vi "Get Data Queue Values.vi"(8 "error in (no error)":errorcluster, 11 "Sift Client in":refnum<class "Sift Client.lvclass">) -> (0 "error out":errorcluster, 2 "map":map{string, variant}(c390), 3 "Sift Client out":refnum<class "Sift Client.lvclass">)   [LabVIEW 2024, in "Sift Client.lvlib" / "Sift Client.lvclass"]
uses:
  Sift Client.lvclass
  Sift Client.lvclass/Sift Client.ctl
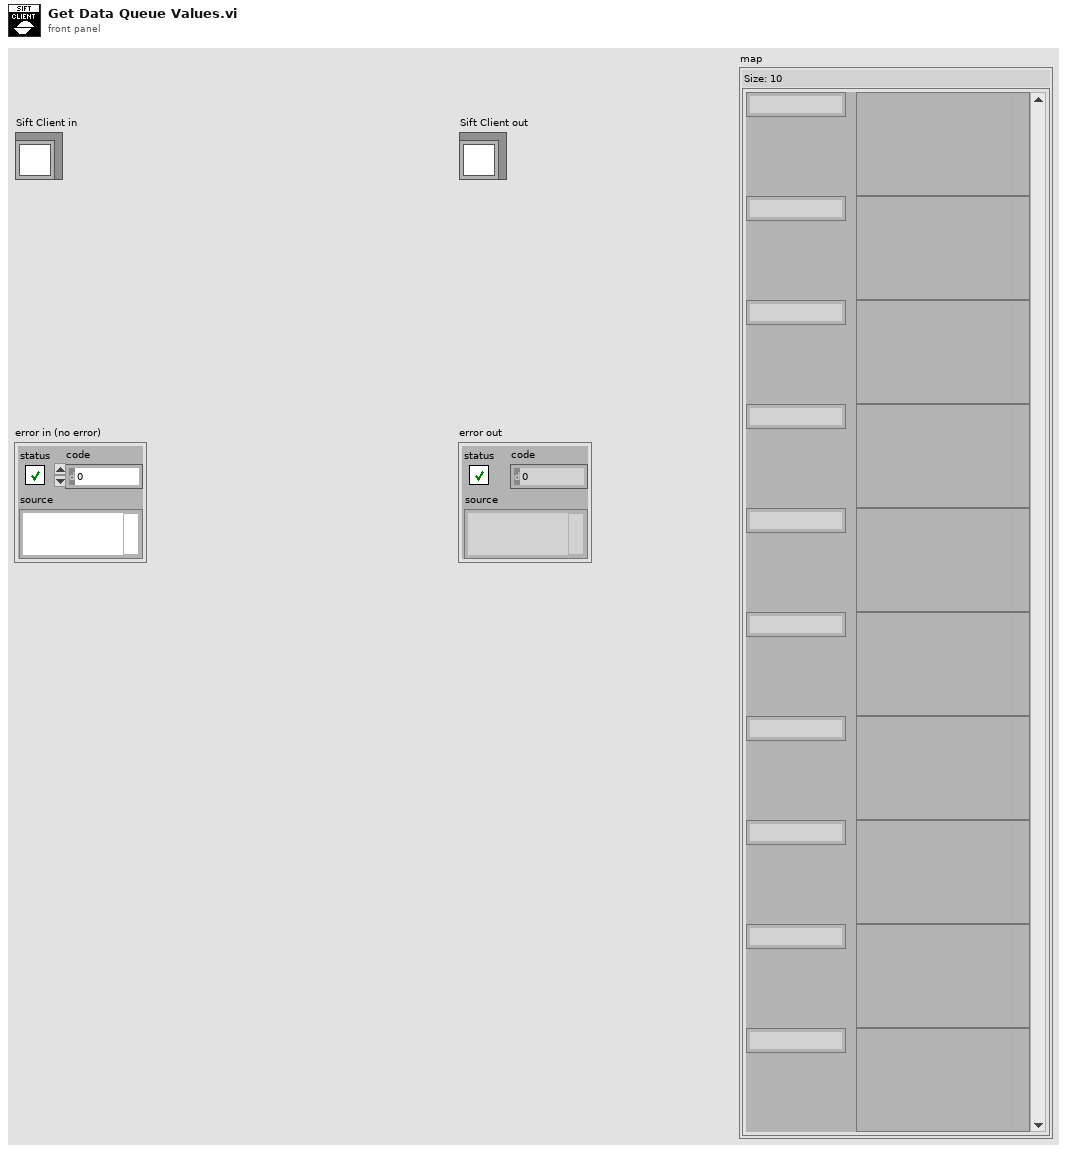
[diagram p1: front panel]
types:
  T1 = typedef "Sift Client.lvlib/String Sample.ctl" = cluster{"Values":string[], "Timestamp":T2, "Flow Name":string}
  T2 = typedef "SiftProxy_client.lvlib/google_protobuf_Timestamp.ctl" = cluster{"seconds":i64, "nanos":i32}
  T3 = typedef "Sift Client.lvlib/Double Sample.ctl" = cluster{"Values":dbl[], "Timestamp":T2, "Flow Name":string}
  T4 = typedef "Sift Client.lvlib/Float Sample.ctl" = cluster{"Values":sgl[], "Timestamp":T2, "Flow Name":string}
  T5 = typedef "Sift Client.lvlib/Int64 Sample.ctl" = cluster{"Values":i64[], "Timestamp":T2, "Flow Name":string}
  T6 = typedef "Sift Client.lvlib/Bool Sample.ctl" = cluster{"Values":bool[], "Timestamp":T2, "Flow Name":string}
  T7 = typedef "Sift Client.lvlib/Int32 Sample.ctl" = cluster{"Values":i32[], "Timestamp":T2, "Flow Name":string}
  T8 = typedef "Sift Client.lvlib/Uint64 Sample.ctl" = cluster{"Values":u64[], "Timestamp":T2, "Flow Name":string}
  T9 = typedef "Sift Client.lvlib/Uint32 Sample.ctl" = cluster{"Values":u32[], "Timestamp":T2, "Flow Name":string}
  T10 = typedef "Sift Client.lvlib/Enum Sample.ctl" = cluster{"Values":u32[], "Timestamp":T2, "Flow Name":string}
  T11 = typedef "Sift Client.lvlib/Bitfield Sample.ctl" = cluster{"Timestamp":T2, "Values":cluster{"Array":u8[]}[], "Flow Name":string}
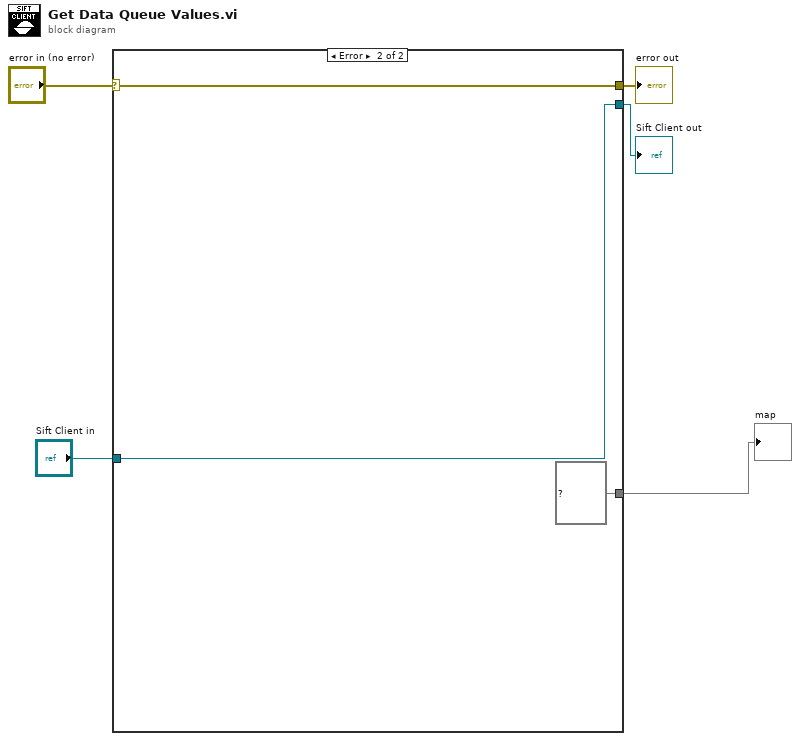
[diagram p0: block diagram]
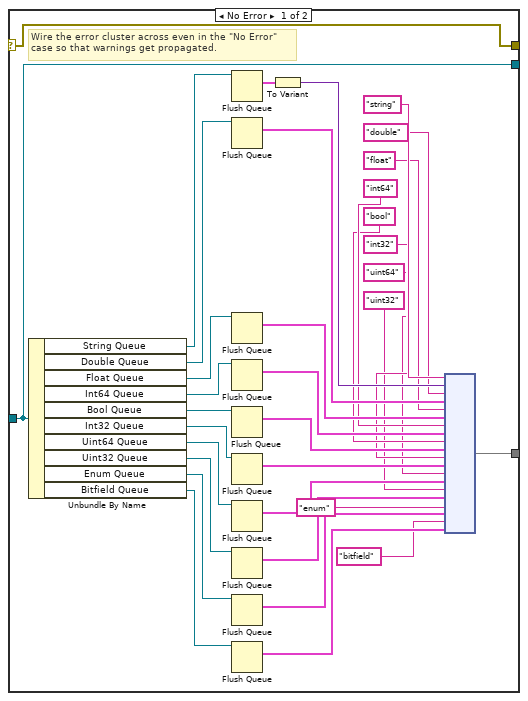
[diagram p2: hidden frame]
diagram:
  n1 = case shown="Error" "error in (no error)" {
    selector: "error in (no error)" -> [w39 w42]
    tunnel: [w39 w42] -> w4
    tunnel: [w38 w41] -> w2
    tunnel: "Sift Client in" -> [w38 w41]
    tunnel: [w6 map{string, variant} {} ("map")] -> w1
    frame No Error {
      # "Wire the error cluster across even in the \"No Error\"\ncase so that warnings get propagated."
      n2 = Unbundle By Name(w38) -> ("String Queue"=w37:refnum<queue>, "Double Queue"=w36:refnum<queue>, "Float Queue"=w35:refnum<queue>, "Int64 Queue"=w34:refnum<queue>, "Bool Queue"=w33:refnum<queue>, "Int32 Queue"=w32:refnum<queue>, "Uint64 Queue"=w31:refnum<queue>, "Uint32 Queue"=w30:refnum<queue>, "Enum Queue"=w29:refnum<queue>, "Bitfield Queue"=w28:refnum<queue>)
      n3 = Flush Queue(queue=w37) -> (remaining elements=w27:T1[])  [unwired: 1 in, 2 out]
      n4 = Flush Queue(queue=w36) -> (remaining elements=w25:T3[])  [unwired: 1 in, 2 out]
      n5 = Flush Queue(queue=w35) -> (remaining elements=w24:T4[])  [unwired: 1 in, 2 out]
      n6 = Flush Queue(queue=w34) -> (remaining elements=w23:T5[])  [unwired: 1 in, 2 out]
      n7 = Flush Queue(queue=w33) -> (remaining elements=w22:T6[])  [unwired: 1 in, 2 out]
      n8 = Flush Queue(queue=w32) -> (remaining elements=w21:T7[])  [unwired: 1 in, 2 out]
      n9 = Flush Queue(queue=w31) -> (remaining elements=w20:T8[])  [unwired: 1 in, 2 out]
      n10 = Flush Queue(queue=w30) -> (remaining elements=w19:T9[])  [unwired: 1 in, 2 out]
      n11 = Flush Queue(queue=w29) -> (remaining elements=w18:T10[])  [unwired: 1 in, 2 out]
      n12 = Flush Queue(queue=w28) -> (remaining elements=w17:T11[])  [unwired: 1 in, 2 out]
      n13 = To Variant(anything=w27) -> (Variant=w26:variant)
      n14 = node("string", w26, "double", w25, "float", w24, "int64", w23, "bool", w22, "int32", w21, "uint64", w20, "uint32", w19, "enum" ("key"), w18, "bitfield" ("key"), w17) -> (w6:map{string, variant})
    }
    frame Error {
    }
  }
  "error out" <- w4
  "Sift Client out" <- w2
  "map" <- w1
